vi "Destroy.vi"(0 "reference in":refnum<class "Select.lvclass">, 5 "error in (no error)":errorcluster) -> (14 "reference out":refnum<class "Select.lvclass">, 19 "error out":errorcluster)   [LabVIEW 2014, in "Select.lvclass"]
uses:
  Select.lvclass
  Control_class/Control.lvclass
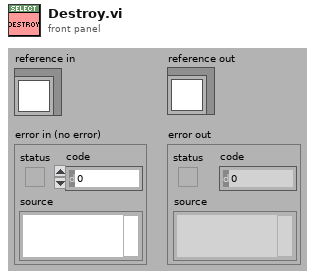
[diagram p1: front panel]
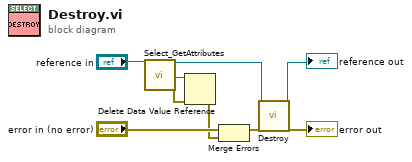
[diagram p0: block diagram]
diagram:
  n1 = call "Select_GetAttributes.vi"("reference in"="reference in") -> ("reference out"=w4:refnum<class "Select.lvclass">, "DataRef"=w7:refnum<data-value>, "error out"=w8:errorcluster)  [unwired: 15 in, 1 out]
  n2 = Delete Data Value Reference(data value reference=w7, error in=w8) -> (error out=w1:errorcluster)  [unwired: 1 out]
  n3 = Merge Errors("error in (no error)", w1) -> (w6:errorcluster)
  n4 = call-parent "Destroy.vi"("reference in"=w4, "error in (no error)"=w6) -> ("reference out"=→"reference out":refnum<class "Select.lvclass">, "error out"=→"error out":errorcluster)  [unwired: 16 in]
